vi "parse_bool.vi"   [LabVIEW 2012]
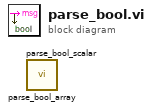
[diagram p0: block diagram]
diagram:
  n1 = call "parse_bool_array.vi"() -> ()  [unwired: 5 in, 3 out]
  n2 = call "parse_bool_scalar.vi"() -> ()  [unwired: 5 in, 3 out]
